vi "Get all project item strings.vi"(8 "error in (no error)":errorcluster, 11 "Project.Reference":refnum<vi>) -> (0 "error out":errorcluster, 2 "All Strings":string[](array[string]))   [LabVIEW 2018, in "Covers-o-meter.lvlib"]
uses:
  Covers-o-meter.lvlib
  <vilib>/Utility/traverseref.llb/TRef TravTarget.ctl
  <vilib>/Utility/traverseref.llb/VI Scripting - Traverse.lvlib
panel:
  out "Control Desc":string[](array[string])
  out "control descriptions":string[](array[string])
  out "Free labels, text (decorations)":string[](array[string])
  out "Class Desc":string[](array[string])
  out "Library desc":string[](array[string])
  out "Descriptions":string[](array[string])
  out "VIs":string[](array[string])
  in  "project":refnum<vi>
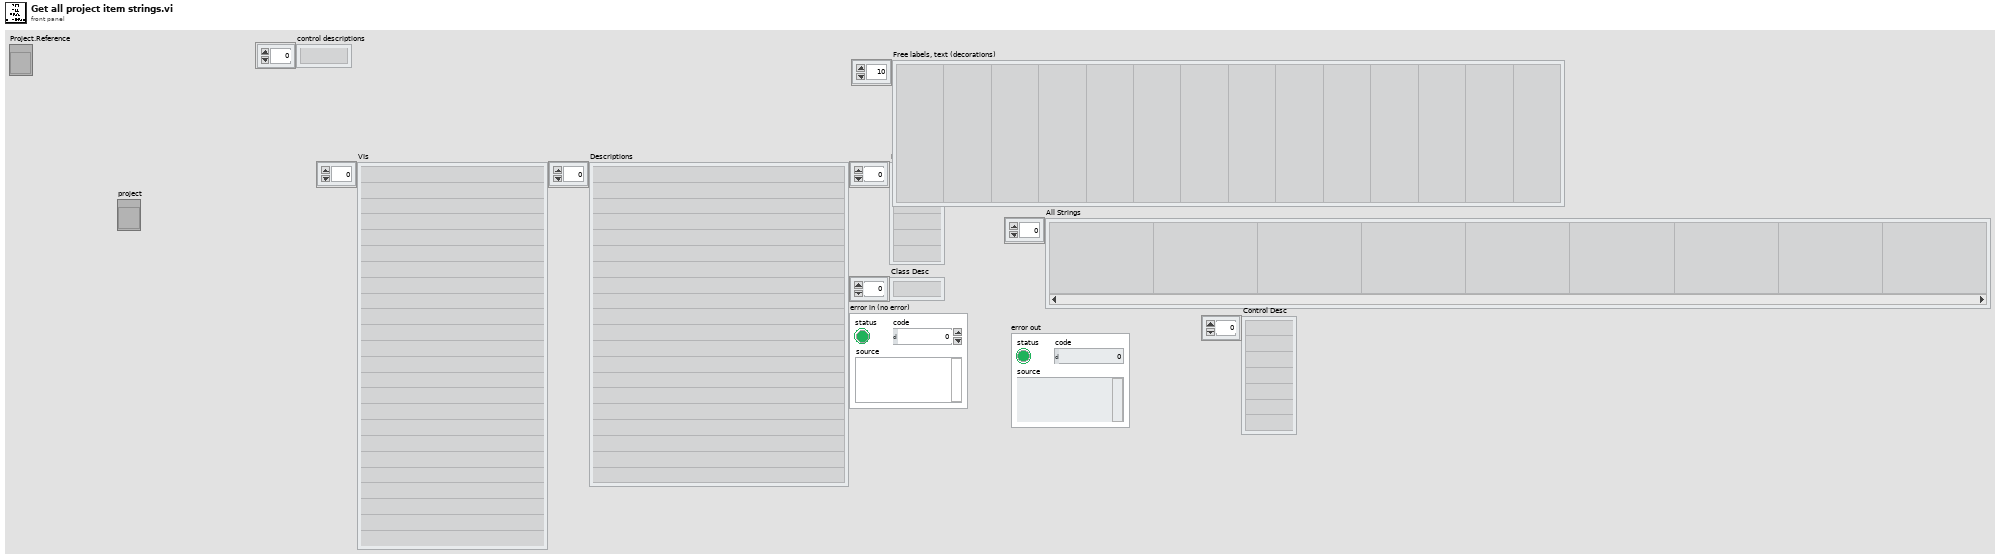
[diagram p1: front panel]
types:
  T1 = typedef "TRef TravTarget.ctl" = enum16{"FP", "BD", "Other"}
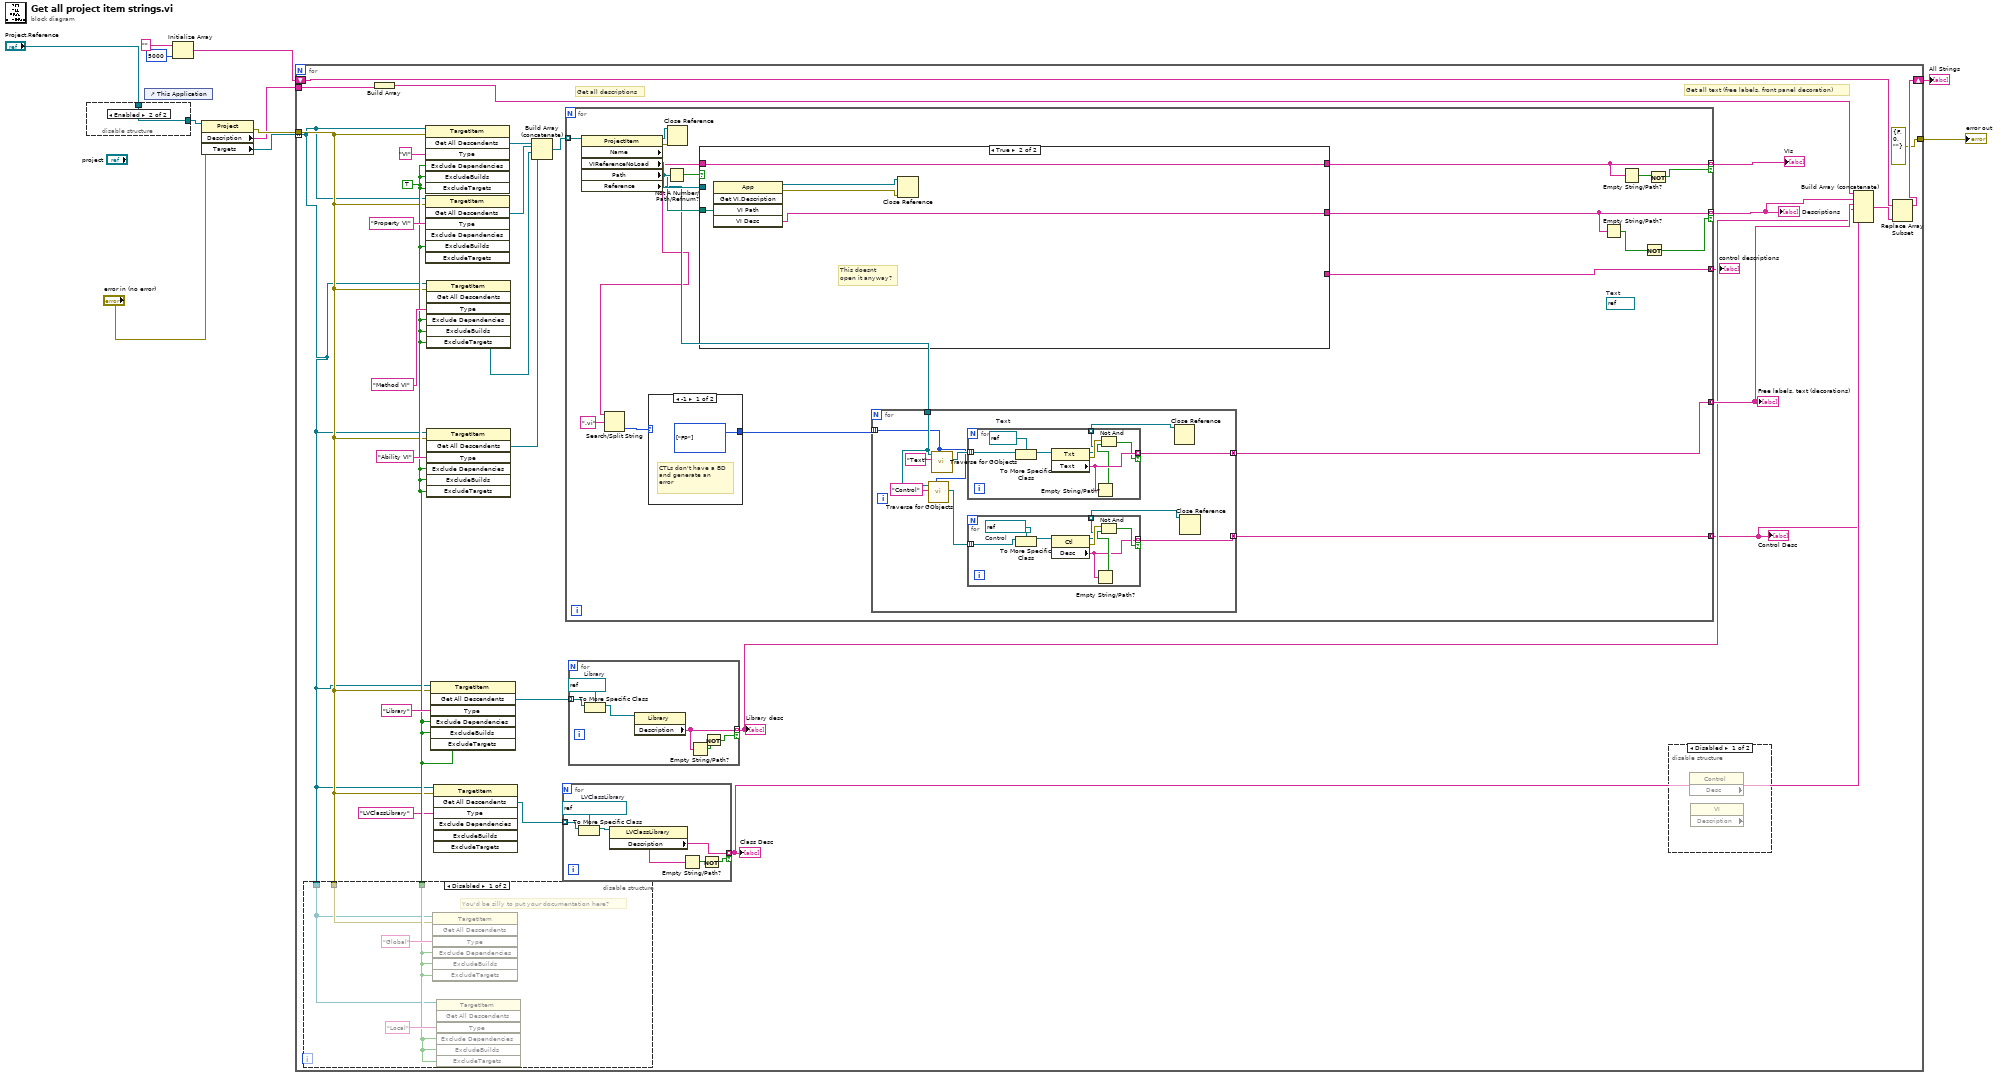
[diagram p0: block diagram]
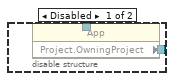
[diagram p2: hidden frame]
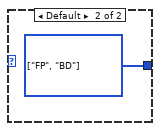
[diagram p4: hidden frame]
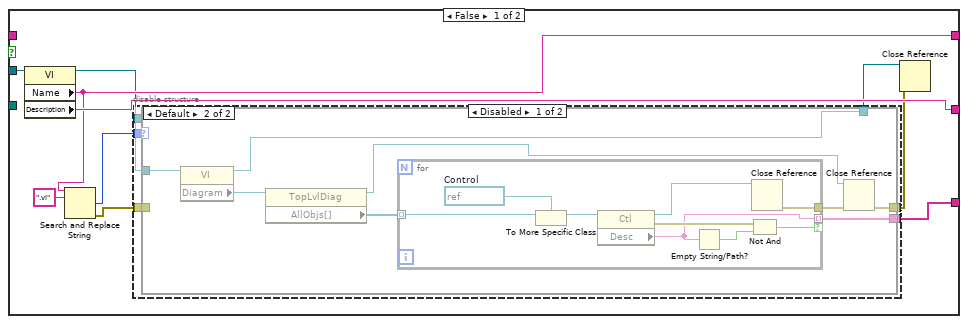
[diagram p5: hidden frame]
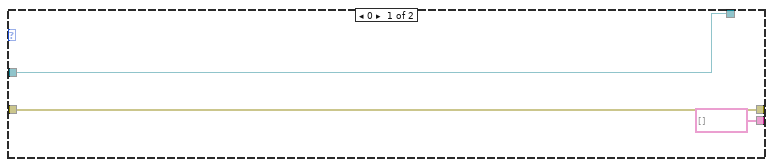
[diagram p6: hidden frame]
diagram:
  n1 = disable-structure shown="Enabled" {
    disable-tunnel: [w12 w13] -> w10
    disable-tunnel: "Project.Reference" -> [_ w13]
    frame Disabled {
      n2 = property class="App"() -> ("Project.OwningProject"=w12:refnum<vi>)  [unwired: 2 in, 2 out]
    }
    frame Enabled {
    }
  }
  n3 = control-ref of="This Application"() -> ()  [unwired: 1 out]
  n4 = Initialize Array("", 5000 ("dimension size")) -> (w5:string[])
  n5 = property class="Project"(reference=w10, error in="error in (no error)") -> (error out=w11:errorcluster, "Description"=w8:string, "Targets"=w9:refnum<vi>[])  [unwired: 1 out]
  n6 = for {
    tunnel: w9 -> [w34] mode=indexing
    tunnel: w11 -> [w35]
    tunnel: w8 -> [w23]
    shift-right: [w18] -> w4
    shift-left: w5 -> [w19]
    tunnel: [errorcluster {"status"=FALSE, "code"=0, "source"=""} ("error constant")] -> w2
    w37 = TRUE ("ExcludeDependencies")
    # "Get all text (free labels, front panel decoration)"
    # "Get all descriptions"
    n7 = disable-structure shown="Disabled" {
      disable-tunnel: w37 -> [w147 _]
      disable-tunnel: w35 -> [w146 _]
      disable-tunnel: w34 -> [w145 _]
      frame Disabled {
        # "You'd be silly to put your documentation here?"
        n8 = invoke class="TargetItem" method="Get All Descendents"(reference=w145, error in=w146, "Type"="Global", "Exclude Dependencies"=w147, "ExcludeBuilds"=w147, "ExcludeTargets"=w147) -> ()  [unwired: 1 in, 7 out]
        n9 = invoke class="TargetItem" method="Get All Descendents"(reference=w145, "Type"="Local", "Exclude Dependencies"=w147, "ExcludeBuilds"=w147, "ExcludeTargets"=w147) -> ()  [unwired: 2 in, 7 out]
      }
      frame Enabled {
      }
    }
    n10 = Build Array(w23) -> (w22:string[])
    n11 = invoke class="TargetItem" method="Get All Descendents"(reference=w34, error in=w35, "Type"="VI", "Exclude Dependencies"=w37, "ExcludeBuilds"=w37, "ExcludeTargets"=w37) -> ("All Descendents"=w33:refnum<vi>[])  [unwired: 1 in, 6 out]
    n12 = invoke class="TargetItem" method="Get All Descendents"(reference=w34, error in=w35, "Type"="Property VI", "Exclude Dependencies"=w37, "ExcludeBuilds"=w37, "ExcludeTargets"=w37) -> ("All Descendents"=w32:refnum<vi>[])  [unwired: 1 in, 6 out]
    n13 = invoke class="TargetItem" method="Get All Descendents"(reference=w34, error in=w35, "Type"="Method VI", "Exclude Dependencies"=w37, "ExcludeBuilds"=w37, "ExcludeTargets"=w37) -> ("All Descendents"=w30:refnum<vi>[])  [unwired: 1 in, 6 out]
    n14 = invoke class="TargetItem" method="Get All Descendents"(reference=w34, error in=w35, "Type"="Ability VI", "Exclude Dependencies"=w37, "ExcludeBuilds"=w37, "ExcludeTargets"=w37) -> ("All Descendents"=w29:refnum<vi>[])  [unwired: 1 in, 6 out]
    n15 = invoke class="TargetItem" method="Get All Descendents"(reference=w34, error in=w35, "Type"="Library", "Exclude Dependencies"=w37, "ExcludeBuilds"=w37, "ExcludeTargets"=w37) -> ("All Descendents"=w28:refnum<vi>[])  [unwired: 1 in, 6 out]
    n16 = invoke class="TargetItem" method="Get All Descendents"(reference=w34, error in=w35, "Type"="LVClassLibrary") -> ("All Descendents"=w27:refnum<vi>[])  [unwired: 4 in, 6 out]
    n17 = Build Array (concatenate)(w33, w32, w30, w29) -> (w31:refnum<vi>[])
    n18 = for {
      tunnel: w27 -> [w138] mode=indexing
      tunnel: [w135] -> w20 mode=indexing if=w133
      w137 = refnum<vi> refnum  # LVClassLibrary
      n19 = To More Specific Class(target class=w137, reference=w138) -> (specific class reference=w136:refnum<vi>)  [unwired: 1 in, 1 out]
      n20 = property class="LVClassLibrary"(reference=w136) -> ("Description"=w135:string)  [unwired: 1 in, 2 out]
      n21 = Empty String/Path?(string/path=w135) -> (empty?=w134:bool)
      n22 = Not(x=w134) -> (.not. x?=w133:bool)
    }
    "Class Desc" <- w20
    n23 = for {
      tunnel: w31 -> [w58] mode=indexing
      tunnel: [w49] -> w26 mode=indexing if=w47
      tunnel: [w50] -> w25 mode=indexing if=w45
      tunnel: [w54] -> w24 mode=concatenating
      tunnel: [w44] -> w15 mode=concatenating
      tunnel: [w43] -> w14 mode=concatenating
      (unwired) refnum<vi> refnum  # Text
      n24 = property class="ProjectItem"(reference=w58) -> (reference out=w61:refnum<vi>, error out=w62:errorcluster, "Name"=w51:string, "VIReferenceNoLoad"=w59:refnum<vi>, "Path"=w57:path, "Reference"=w55:refnum<vi>)  [unwired: 1 in]
      n25 = Search/Split String(string=w51, search string/char (-)=".vi") -> (offset of match=w52:i32)  [unwired: 1 in, 2 out]
      n26 = case shown="-1" w52 {
        tunnel: [w63 w64] -> w56
        frame -1 {
          w63 = T1[] [enum."FP"] items=["FP", "BD", "Other"]
          # "CTLs don't have a BD\nand generate an \nerror"
        }
        frame Default {
          w64 = T1[] [enum."FP", enum."BD"] items=["FP", "BD", "Other"]
        }
      }
      n27 = Not A Number/Path/Refnum?(number/path/refnum=w59) -> (NaN/Path/Refnum?=w60:bool)
      n28 = Close Reference(reference=w61, error in (no error)=w62) -> ()  [unwired: 1 out]
      n29 = case shown="True" w60 {
        tunnel: w51 -> [_ w132]
        tunnel: [w97 w132] -> w49
        tunnel: w59 -> [w100 _]
        tunnel: [w99 w130] -> w50
        tunnel: w57 -> [_ w131]
        tunnel: [w98 _] -> w44
        frame False {
          n30 = property class="VI"(reference=w100) -> (reference out=w92:refnum<vi>, "Name"=w97:string, "Description"=w99:string)  [unwired: 1 in, 1 out]
          n31 = Search and Replace String(input string=w97, search string=".vi") -> (number of replacements=w94:i32, error out=w93:errorcluster)  [unwired: 6 in, 2 out]
          n32 = disable-structure shown="Disabled" {
            disable-tunnel: [w106 _] -> w98
            disable-tunnel: [w105 _] -> w95
            disable-tunnel: w94 -> [w104 _]
            disable-tunnel: w93 -> [w103 _]
            disable-tunnel: w92 -> [w102 w127]
            disable-tunnel: [w101 w127] -> w91
            frame Disabled {
              n33 = case shown="Default" w104 {
                tunnel: [string[] [] w116] -> w106
                tunnel: [w109 w111] -> w105
                tunnel: w103 -> [w109 _]
                tunnel: w102 -> [w108 w115]
                tunnel: [w108 w113] -> w101
                frame 0 {
                }
                frame Default {
                  n34 = property class="VI"(reference=w115) -> (reference out=w113:refnum<vi>, "Diagram"=w114:refnum<vi>)  [unwired: 1 in, 1 out]
                  n35 = property class="TopLvlDiag"(reference=w114) -> (reference out=w110:refnum<vi>, "AllObjs[]"=w117:refnum<vi>[])  [unwired: 1 in, 1 out]
                  n36 = for {
                    tunnel: w117 -> [w126] mode=indexing
                    tunnel: [w121] -> w116 mode=indexing if=w120
                    tunnel: [w118] -> w112
                    w125 = refnum<vi> refnum  # Control
                    n37 = To More Specific Class(target class=w125, reference=w126) -> (specific class reference=w124:refnum<vi>)  [unwired: 1 in, 1 out]
                    n38 = property class="Ctl"(reference=w124) -> (reference out=w119:refnum<vi>, error out=w122:errorcluster, "Desc"=w121:string)  [unwired: 1 in]
                    n39 = Empty String/Path?(string/path=w121) -> (empty?=w123:bool)
                    n40 = Not And(1:w123, 2:w122) -> (0:w120:bool)
                    n41 = Close Reference(reference=w119) -> (error out=w118:errorcluster)  [unwired: 1 in]
                  }
                  n42 = Close Reference(reference=w110, error in (no error)=w112) -> (error out=w111:errorcluster)
                }
              }
            }
            frame Enabled {
            }
          }
          n43 = Close Reference(reference=w91, error in (no error)=w95) -> ()  [unwired: 1 out]
        }
        frame True {
          # "This doesnt \nopen it anyway?"
          n44 = invoke class="App" method="Get VI.Description"("VI Path"=w131) -> (reference out=w129:refnum<vi>, error out=w128:errorcluster, "VI Desc"=w130:string)  [unwired: 4 in, 2 out]
          n45 = Close Reference(reference=w129, error in (no error)=w128) -> ()  [unwired: 1 out]
        }
      }
      n46 = for {
        tunnel: [w72] -> w54 mode=concatenating
        tunnel: w56 -> [w67] mode=indexing
        tunnel: w55 -> [w71]
        tunnel: [w68] -> w43 mode=concatenating
        n47 = call <vilib>:"Traverse for GObjects.vi"("Traverse Target"=w67, "Class Name"="Control", "VI Refnum"=w71) -> ("References"=w69:refnum<vi>[])  [unwired: 5 in, 3 out]
        n48 = call <vilib>:"Traverse for GObjects.vi"("Traverse Target"=w67, "Class Name"="Text", "VI Refnum"=w71) -> ("References"=w73:refnum<vi>[])  [unwired: 5 in, 3 out]
        n49 = for {
          tunnel: w73 -> [w90] mode=indexing
          tunnel: [w87] -> w72 mode=indexing if=w84
          tunnel: [w83] -> w66 mode=indexing
          w88 = refnum<vi> refnum  # Text
          n50 = To More Specific Class(target class=w88, reference=w90) -> (specific class reference=w89:refnum<vi>)  [unwired: 1 in, 1 out]
          n51 = property class="Txt"(reference=w89) -> (reference out=w83:refnum<vi>, error out=w85:errorcluster, "Text"=w87:string)  [unwired: 1 in]
          n52 = Empty String/Path?(string/path=w87) -> (empty?=w86:bool)
          n53 = Not And(1:w86, 2:w85) -> (0:w84:bool)
        }
        n54 = for {
          tunnel: [w76] -> w68 mode=indexing if=w79
          tunnel: w69 -> [w77] mode=indexing
          tunnel: [w75] -> w65 mode=indexing
          w78 = refnum<vi> refnum  # Control
          n55 = To More Specific Class(target class=w78, reference=w77) -> (specific class reference=w82:refnum<vi>)  [unwired: 1 in, 1 out]
          n56 = property class="Ctl"(reference=w82) -> (reference out=w75:refnum<vi>, error out=w80:errorcluster, "Desc"=w76:string)  [unwired: 1 in]
          n57 = Empty String/Path?(string/path=w76) -> (empty?=w81:bool)
          n58 = Not And(1:w81, 2:w80) -> (0:w79:bool)
        }
        n59 = Close Reference(reference=w66) -> ()  [unwired: 1 in, 1 out]
        n60 = Close Reference(reference=w65) -> ()  [unwired: 1 in, 1 out]
      }
      n61 = Empty String/Path?(string/path=w50) -> (empty?=w46:bool)
      n62 = Empty String/Path?(string/path=w49) -> (empty?=w48:bool)
      n63 = Not(x=w46) -> (.not. x?=w45:bool)
      n64 = Not(x=w48) -> (.not. x?=w47:bool)
    }
    "VIs" <- w26
    "Descriptions" <- w25
    "Free labels, text (decorations)" <- w24
    "control descriptions" <- w15
    "Control Desc" <- w14
    n65 = for {
      tunnel: w28 -> [w144] mode=indexing
      tunnel: [w141] -> w21 mode=indexing if=w139
      w143 = refnum<vi> refnum  # Library
      n66 = To More Specific Class(target class=w143, reference=w144) -> (specific class reference=w142:refnum<vi>)  [unwired: 1 in, 1 out]
      n67 = property class="Library"(reference=w142) -> ("Description"=w141:string)  [unwired: 1 in, 2 out]
      n68 = Empty String/Path?(string/path=w141) -> (empty?=w140:bool)
      n69 = Not(x=w140) -> (.not. x?=w139:bool)
    }
    "Library desc" <- w21
    n70 = disable-structure shown="Disabled" {
      frame Disabled {
        n71 = property class="Control" props=["Desc"]() -> ()  [unwired: 2 in, 3 out]
        n72 = property class="VI" props=["Description"]() -> ()  [unwired: 2 in, 3 out]
      }
      frame Enabled {
      }
    }
    n73 = Build Array (concatenate)(w22, w25, w24, w21, w20, w14) -> (w16:string[])
    n74 = Replace Array Subset(array=w19, new element=w16) -> (w18:string[])  [unwired: 1 in]
  }
  "All Strings" <- w4
  "error out" <- w2
